vi "ULx Write (Digital Wfm 1Chan NSamp).vi"(0 "task in":refnum<k24>, 1 "auto start":bool, 7 "data":digitalwaveform(waveform)={"t0"=timestamp(0 s since 1904-01-01), "dt"=0.0, "Y"={"transitions"=[], "data"=[]}, "error"={"status"=FALSE, "code"=37421928, "source"=""}}, 9 "timeout":dbl=10.0 format="%_4g", 11 "error in":errorcluster) -> (4 "task out":refnum<k24>, 10 "number of samples written per channel":u32, 15 "error out":errorcluster)   [LabVIEW 2020]
doc: "Writes a digital waveform to a task that contains a single digital output channel."
uses:
  C:/Users/William/Documents/LV 2020 builds/LeaktestDAQ/Source-v33/ULx_LV.dll
  ULx_LV.dll
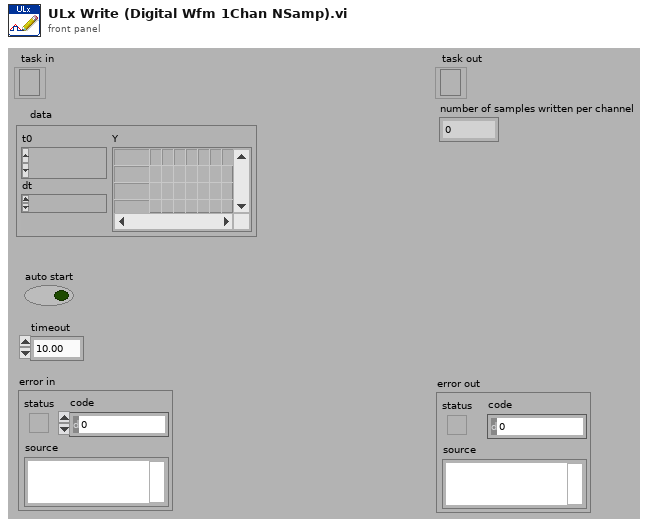
[diagram p1: front panel]
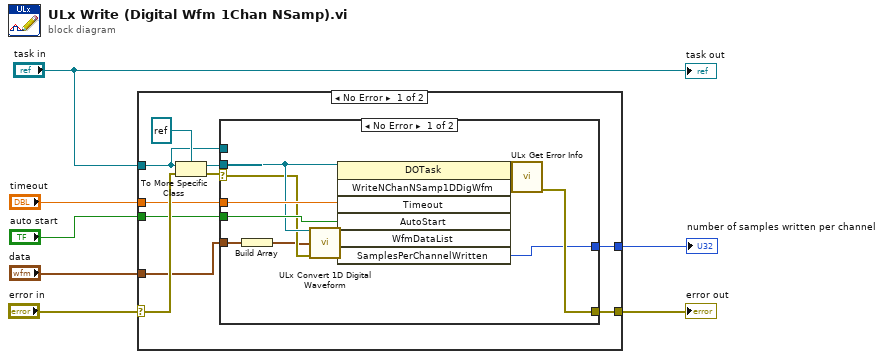
[diagram p0: block diagram]
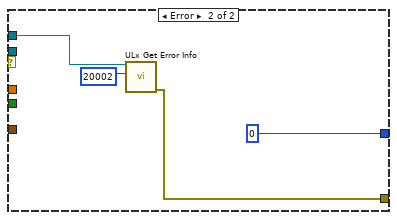
[diagram p2: hidden frame]
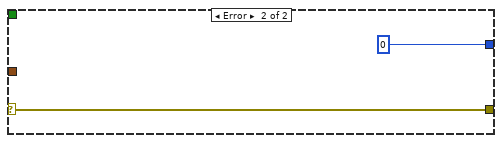
[diagram p3: hidden frame]
diagram:
  n1 = case shown="No Error" "error in" {
    selector: "error in" -> [w17 w35]
    tunnel: "task in" -> [w11 _]
    tunnel: "timeout" -> [w13 _]
    tunnel: [w12 w35] -> w5
    tunnel: "auto start" -> [w10 _]
    tunnel: [w9 0 ("SamplesPerChannelWritten")] -> w2
    tunnel: "data" -> [w8 _]
    frame No Error {
      n2 = To More Specific Class(target class=refnum<k24> refnum, reference=w11, error in=w17) -> (specific class reference=w14:refnum<k24>, error out=w15:errorcluster)
      n3 = case shown="No Error" w15 {
        selector: w15 -> [w24 _]
        tunnel: w14 -> [w25 _]
        tunnel: w13 -> [w27 _]
        tunnel: [w29 w32] -> w12
        tunnel: w11 -> [_ w31]
        tunnel: w10 -> [w26 _]
        tunnel: [w28 0 ("SamplesPerChannelWritten")] -> w9
        tunnel: w8 -> [w23 _]
        frame No Error {
          n4 = Build Array(w23) -> (w19:digitalwaveform[])
          n5 = call "ULx Convert 1D Digital Waveform.vi"("task in"=w25, "data"=w19, "error in"=w24) -> ("data List"=w18:refnum<k24>)  [unwired: 11 in, 1 out]
          n6 = invoke class="DOTask" method="WriteNChanNSamp1DDigWfm"(reference=w25, "Timeout"=w27, "AutoStart"=w26, "WfmDataList"=w18) -> (reference out=w21:refnum<k24>, error out=w22:errorcluster, "WriteNChanNSamp1DDigWfm"=w20:i32, "SamplesPerChannelWritten"=w28:u32)  [unwired: 3 in, 3 out]
          n7 = call "ULx Get Error Info.vi"("error in"=w22, "ErrorCode"=w20, "task in"=w21) -> ("error out"=w29:errorcluster)  [unwired: 8 in]
        }
        frame Error {
          n8 = call "ULx Get Error Info.vi"("ErrorCode"=20002, "task in"=w31) -> ("error out"=w32:errorcluster)  [unwired: 9 in]
        }
      }
    }
    frame Error {
    }
  }
  "error out" <- w5
  "number of samples written per channel" <- w2
  "task out" <- "task in"
